vi "Allan Variance.vi"(8 "error in (no error)":errorcluster, 9 "n":u32, 10 "Frequency (Hz)":u32=200, 11 "Data in":dbl[](array[numeric])) -> (0 "error out":errorcluster, 1 "actual sample time (s)":dbl, 2 "Allan Variance":dbl)   [LabVIEW 2021, in "IMU Processing.lvlib"]
uses:
  IMU Processing.lvlib
  <vilib>/Utility/error.llb/DialogType.ctl
panel:
  out "max index(es)":i32
  out "max value":dbl
  out "sum":dbl
  out "Numeric":dbl
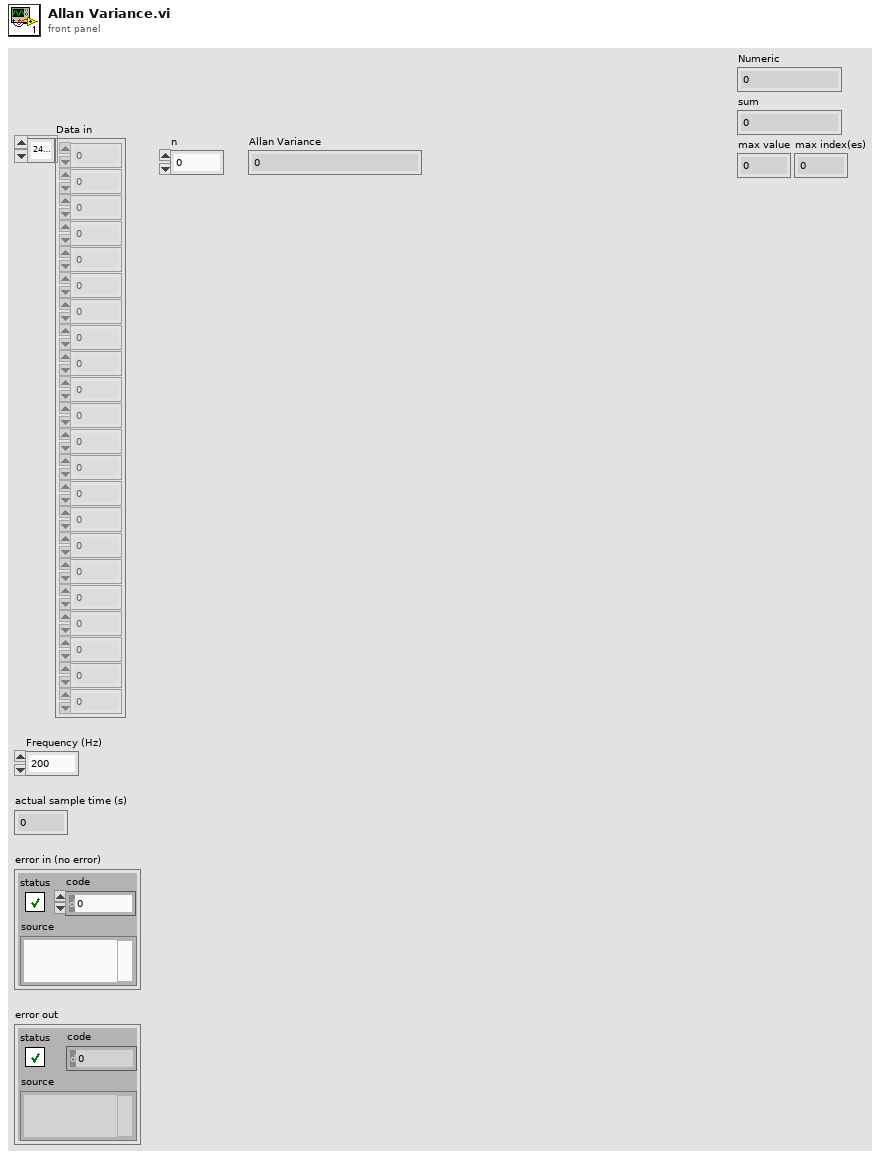
[diagram p1: front panel]
types:
  T1 = typedef "DialogType.ctl" = u16
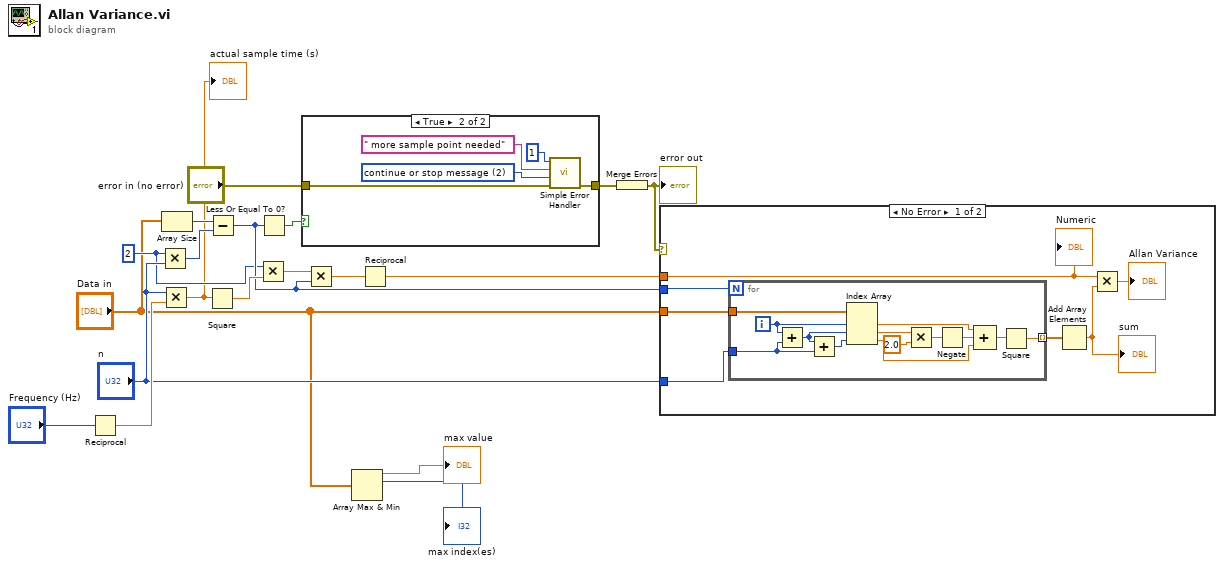
[diagram p0: block diagram]
diagram:
  w6 = 2 ("x")
  n1 = Reciprocal(x="Frequency (Hz)") -> (1/x=w14:dbl)
  n2 = Multiply(x=w6, y="n") -> (x*y=w12:u32)
  n3 = Multiply(x="n", y=w14) -> (x*y=w4:dbl)
  "actual sample time (s)" <- w4
  n4 = Array Size(array="Data in") -> (size(s)=w13:i32)
  n5 = Square(x=w4) -> (x^2=w11:dbl)
  n6 = Subtract(x=w13, y=w12) -> (x-y=w9:u32)
  n7 = Multiply(x=w6, y=w11) -> (x*y=w10:dbl)
  n8 = Less Or Equal To 0?(x=w9) -> (x <= 0?=w19:bool)
  n9 = case shown="True" w19 {
    tunnel: "error in (no error)" -> [w20 w25]
    tunnel: [w20 w24] -> w18
    frame False {
    }
    frame True {
      w22 = T1 2 items=["no dialog", "OK message", "continue or stop message", "OK message + warnings", "continue/stop + warnings"] ("type of dialog (OK msg:1)")
      n10 = call <vilib>:"Simple Error Handler.vi"("error code (no error:0)"=1, "error source (\" \")"=" more sample point needed" ("error source (\" \")"), "type of dialog (OK msg:1)"=w22, "error in (no error)"=w25) -> ("error out"=w24:errorcluster)  [unwired: 1 in, 4 out]
    }
  }
  n11 = Multiply(x=w10, y=w9) -> (x*y=w8:dbl)
  n12 = Array Max & Min(array="Data in") -> (max value=→"max value":dbl, max index (indices)=→"max index(es)":i32)  [unwired: 2 out]
  n13 = Reciprocal(x=w8) -> (1/x=w5:dbl)
  n14 = Merge Errors(w18) -> (w16:errorcluster)
  "error out" <- w16
  n15 = case shown="No Error" w16 {
    tunnel: w9 -> [w32 _]
    tunnel: "Data in" -> [w31 _]
    tunnel: "n" -> [w30 _]
    tunnel: w5 -> [w27 _]
    frame No Error {
      n16 = for {
        N: w32 -> [_]
        tunnel: w31 -> [w40]
        tunnel: w30 -> [w42]
        tunnel: [w33] -> w29 mode=indexing
        i -> [w43]
        n17 = Add(x=w43, y=w42) -> (x+y=w44:u32)
        n18 = Add(x=w44, y=w42) -> (x+y=w45:u32)
        n19 = Index Array(array=w40, index #1=w43, index #2=w44, index #3=w45) -> (element #1=w41:dbl, element #2=w39:dbl, element #3=w38:dbl)
        n20 = Multiply(x=w39, y=2.0) -> (x*y=w37:dbl)
        n21 = Negate(x=w37) -> (-x=w35:dbl)
        n22 = Compound Arithmetic op=ADD(w41, w35, w38) -> (w34:dbl)
        n23 = Square(x=w34) -> (x^2=w33:dbl)
      }
      n24 = Add Array Elements(numeric array=w29) -> (sum=w28:dbl)
      "sum" <- w28
      n25 = Multiply(x=w27, y=w28) -> (x*y=→"Allan Variance":dbl)
      "Numeric" <- w27
    }
    frame Error {
    }
  }
